vi "check pulse 2.vi"() -> ()   [LabVIEW 2014]
panel:
  out "out":bool[](array[boolean])
  in  "in":bool[](array[boolean])
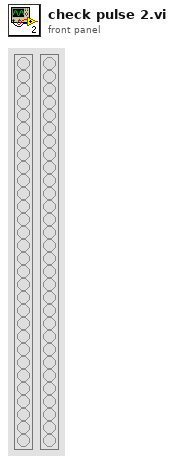
[diagram p1: front panel]
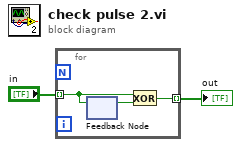
[diagram p0: block diagram]
diagram:
  n1 = for {
    tunnel: "in" -> [w4] mode=indexing
    tunnel: [w3] -> w1 mode=indexing
    n2 = feedback #1() -> (w5:bool)  [unwired: 1 in]
    n3 = feedback-in #1(w4) -> ()
    n4 = Exclusive Or(1:w5, 2:w4) -> (0:w3:bool)
  }
  "out" <- w1
